vi "cw_3_3.vi"() -> ()   [LabVIEW 2022 SP3]
uses:
  <vilib>/numeric/sub_Random U32.vi
  <vilib>/numeric/Random Number (Range) U64.vi
panel:
  in  "K":i32
  out "Array":i32[][](array[numeric])
  in  "M":i32
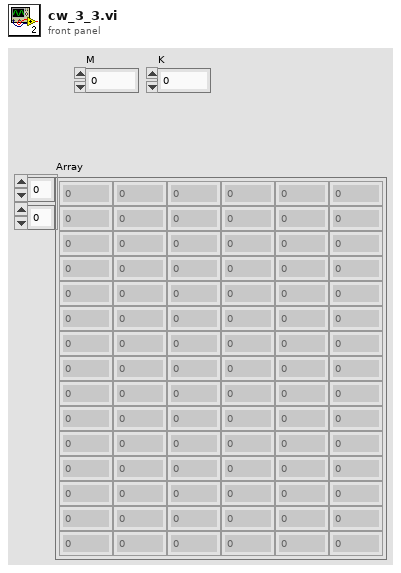
[diagram p1: front panel]
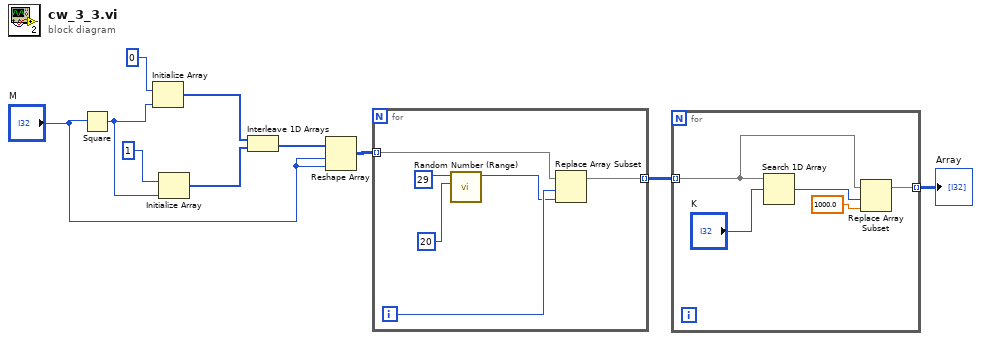
[diagram p0: block diagram]
diagram:
  n1 = Square(x="M") -> (x^2=w5:i32)
  n2 = Initialize Array(0 ("element"), w5) -> (w8:i32[])
  n3 = Initialize Array(1 ("element"), w5) -> (w7:i32[])
  n4 = Interleave 1D Arrays(w8, w7) -> (w6:i32[])
  n5 = Reshape Array(w6, "M", "M") -> (w3:i32[][])
  n6 = for {
    tunnel: w3 -> [w12] mode=indexing
    tunnel: [w11] -> w2 mode=indexing
    i -> [w14]
    n7 = call-poly <vilib>:"Random Number (Range).vi"("lower bound (0)"=u64 20, "upper bound (100)"=u64 29) -> ("number"=w13:u64)  [unwired: 9 in]
    n8 = Replace Array Subset(array=w12, new element=w13, index=w14) -> (w11:i32[])
  }
  n9 = for {
    tunnel: w2 -> [w18] mode=indexing
    tunnel: [w17] -> w1 mode=indexing
    n10 = Search 1D Array(1D array=w18, element="K") -> (index of element=w20:i32)  [unwired: 1 in]
    n11 = Replace Array Subset(array=w18, new element=1000.0 ("new element/subarray"), index=w20) -> (w17:i32[])
  }
  "Array" <- w1
